vi "Close File Transfer Behavior.vi"(8 "error in (no error)":errorcluster, 10 "File Transfer Behavior in":refnum<class "File Transfer Behavior.lvclass">, 11 "RT Management in":refnum<class "RT Management.lvclass">) -> (0 "error out":errorcluster, 3 "RT Management out":refnum<class "RT Management.lvclass">)   [LabVIEW 2016, in "RT Management.lvlib" / "RT Management.lvclass"]
doc: "Closes the File Transfer Behavior, closing out any opened references."
uses:
  RT Management.lvclass
  File Transfer Behavior/File Transfer Behavior.lvclass
  RT Management.lvclass/RT Management.ctl
  Set File Transfer Behavior.lvclass.vi
  Get File Transfer Behavior.lvclass.vi
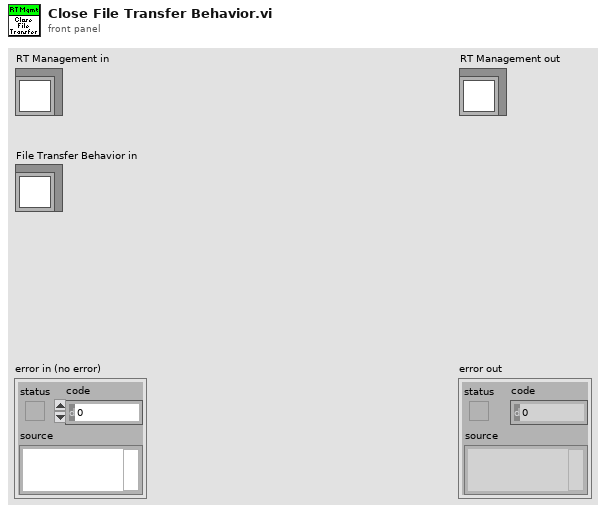
[diagram p1: front panel]
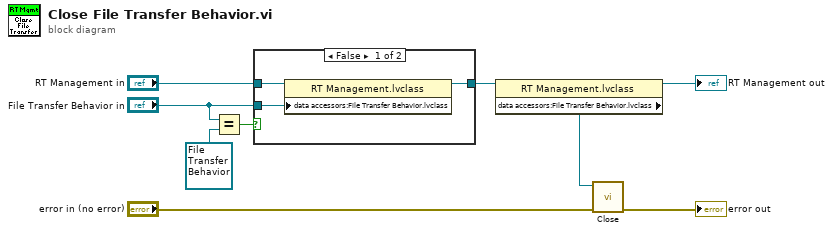
[diagram p0: block diagram]
diagram:
  n1 = Equal?(x="File Transfer Behavior in", y=refnum<class "File Transfer Behavior.lvclass"> refnum ("File Transfer Behavior in")) -> (x = y?=w3:bool)
  n2 = case shown="False" w3 {
    tunnel: "RT Management in" -> [w12 w13]
    tunnel: [w11 w13] -> w5
    tunnel: "File Transfer Behavior in" -> [w10 _]
    frame False {
      n3 = property class="RT Management.lvclass"(reference=w12, "data accessors:File Transfer Behavior.lvclass"=w10) -> (reference out=w11:refnum<class "RT Management.lvclass">)  [unwired: 1 in, 1 out]
    }
    frame True {
    }
  }
  n4 = property class="RT Management.lvclass"(reference=w5) -> (reference out=→"RT Management out":refnum<class "RT Management.lvclass">, "data accessors:File Transfer Behavior.lvclass"=w8:refnum<class "File Transfer Behavior.lvclass">)  [unwired: 1 in, 1 out]
  n5 = call-dynamic "Close.vi"("error in (no error)"="error in (no error)", "File Transfer Behavior in"=w8) -> ("error out"=→"error out":errorcluster)  [unwired: 9 in]
